vi "testRSAEncrypt&DecryptLongData.vi"(8 "error in (no error)":errorcluster, 11 "TestCase in":refnum<class "TestRSA.lvclass">) -> (0 "error out":errorcluster, 3 "TestCase out":refnum<class "TestRSA.lvclass">)   [LabVIEW 2021, in "TestRSA.lvclass"]
uses:
  TestRSA.lvclass
  Asymmetric Encryption/RSA/RSAEncryptionPadding.ctl
  <vilib>/addons/_JKI Toolkits/VI Tester/TestCase.llb/TestCase.lvclass
  Asymmetric Encryption/dotNET Crypto Asymmetric Encryption.lvlib
  Key Management/dotNET Crypto Key Management.lvlib
  C:/Program Files (x86)/National Instruments/LabVIEW 2021/vi.lib/addons/_JKI Toolkits/VI Tester/TestCase.llb/TestCase.lvclass
panel:
  out "length":i32
  out "Decrypted data":string
  out "Encrypted data":string
  out "Encrypted data out":u8[](array[numeric])
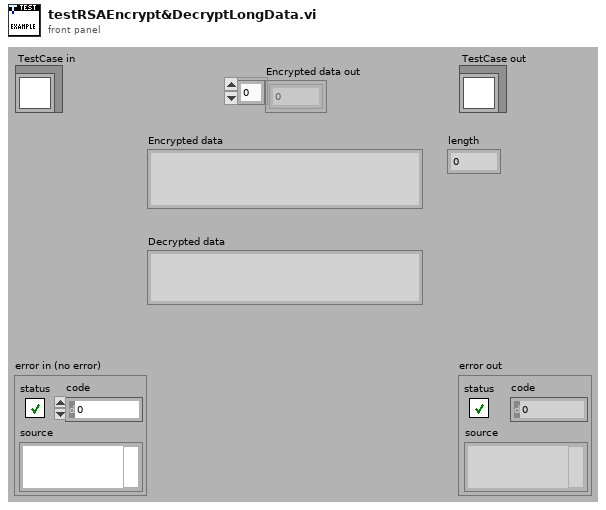
[diagram p1: front panel]
types:
  T1 = typedef "dotNET Crypto Asymmetric Encryption.lvlib/RSAEncryptionPadding.ctl" = enum16{"OaepSHA1", "OaepSHA256", "OaepSHA384", "OaepSHA512", "Pkcs1"}
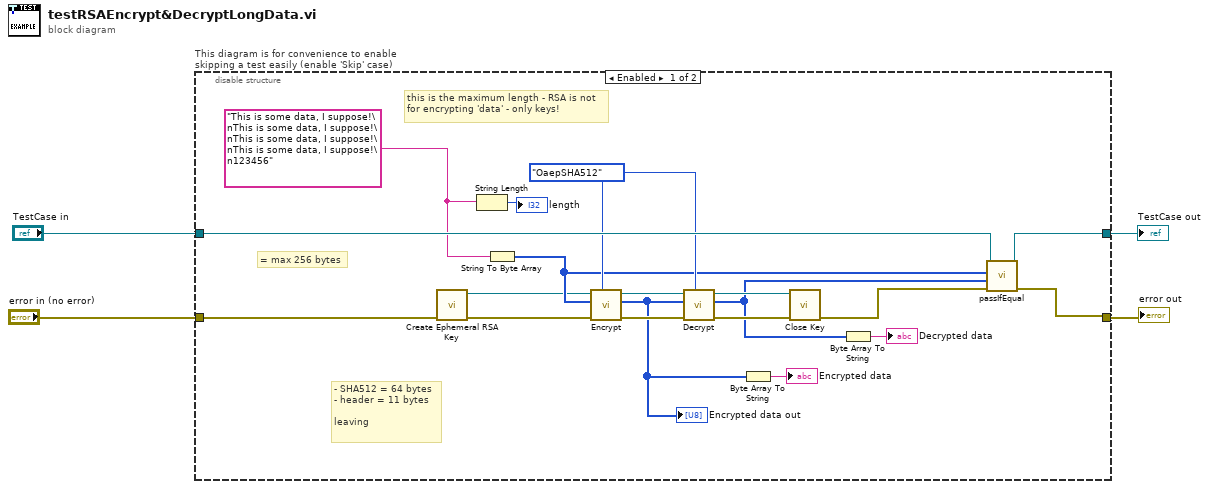
[diagram p0: block diagram]
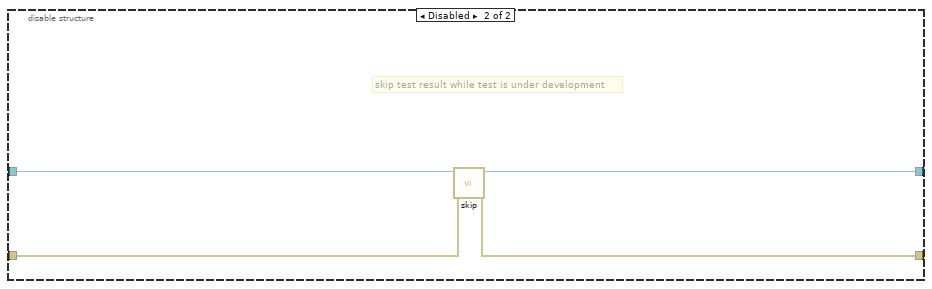
[diagram p2: hidden frame]
diagram:
  n1 = disable-structure "This diagram is for convenience to enable skipping a test easily (enable 'Skip' case)" shown="Enabled" {
    disable-tunnel: "TestCase in" -> [w23 w27]
    disable-tunnel: [w22 w25] -> w1
    disable-tunnel: [w21 w26] -> w3
    disable-tunnel: "error in (no error)" -> [w7 w24]
    frame Enabled {
      w15 = "This is some data, I suppose!\nThis is some data, I suppose!\nThis is some data, I suppose!\nThis is some data, I suppose!\n123456"
      w18 = RSAEncryptionPadding."OaepSHA512" ("Padding Mode")
      # "this is the maximum length - RSA is not for encrypting 'data' - only keys!"
      # "- SHA512 = 64 bytes\n- header = 11 bytes\n\nleaving"
      # "= max 256 bytes"
      n2 = call "Create Ephemeral RSA Key.vi"("error in (no error)"=w7) -> ("error out"=w6:errorcluster, "CngKey out"=w5:refnum<k24>)  [unwired: 9 in]
      n3 = String Length(string=w15) -> (length=→"length":i32)
      n4 = String To Byte Array(string=w15) -> (unsigned byte array=w13:u8[])
      n5 = call "Encrypt.vi"("Padding Mode"=w18, "error in (no error)"=w6, "Raw data in"=w13, "CngKey in"=w5) -> ("error out"=w20:errorcluster, "Encrypted data out"=w11:u8[], "CngKey out"=w12:refnum<k24>)  [unwired: 5 in]
      "Encrypted data out" <- w11
      n6 = call "Decrypt.vi"("Padding Mode"=w18, "error in (no error)"=w20, "Encrypted data in"=w11, "CngKey in"=w12) -> ("error out"=w19:errorcluster, "Raw data out"=w8:u8[], "CngKey out"=w9:refnum<k24>)  [unwired: 5 in]
      n7 = Byte Array To String(unsigned byte array=w11) -> (string=→"Encrypted data":string)
      n8 = call "Close Key.vi"("error in (no error)"=w19, "CngKey in"=w9) -> ("error out"=w10:errorcluster)  [unwired: 9 in]
      n9 = Byte Array To String(unsigned byte array=w8) -> (string=→"Decrypted data":string)
      n10 = call-dynamic "passIfEqual.vi"("error in (no error)"=w10, "y"=w8, "x"=w13, "TestCase in"=w23) -> ("error out"=w21:errorcluster, "TestCase out"=w22:refnum<class "TestRSA.lvclass">)  [unwired: 6 in]
    }
    frame Disabled {
      # "skip test result while test is under development"
      n11 = call <vilib>:"skip.vi"("error in (no error)"=w24, "TestCase in"=w27) -> ("error out"=w26:errorcluster, "TestCase out"=w25:refnum<class "TestRSA.lvclass">)  [unwired: 8 in]
    }
  }
  "error out" <- w3
  "TestCase out" <- w1
